vi "Read From String Format.vi"(8 "error in (no error)":errorcluster, 11 "Numeric in":refnum<class "Abs_Numeric_1D.lvclass">) -> (0 "error out":errorcluster, 2 "From String Format":string="%f", 3 "Numeric out":refnum<class "Abs_Numeric_1D.lvclass">)   [LabVIEW 2021, in "Abs_Numeric_1D.lvclass"]
uses:
  Abs_Numeric_1D.lvclass
  Abs_Numeric_1D.lvclass/Abs_Numeric_1D.ctl
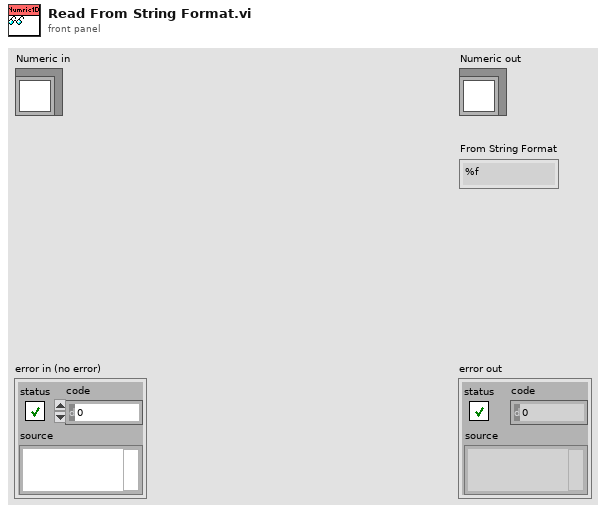
[diagram p1: front panel]
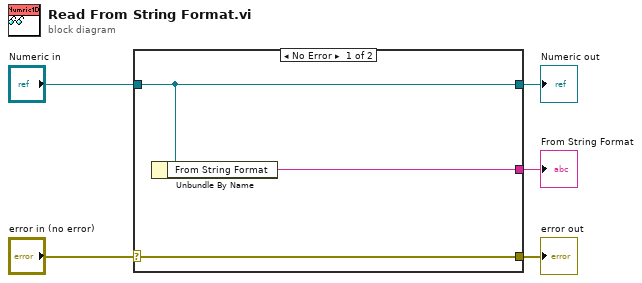
[diagram p0: block diagram]
diagram:
  n1 = case shown="No Error" "error in (no error)" {
    selector: "error in (no error)" -> [w8 w9]
    tunnel: [w8 w9] -> w4
    tunnel: [w7 w10] -> w2
    tunnel: "Numeric in" -> [w7 w10]
    tunnel: [w6 _] -> w1
    frame No Error {
      n2 = Unbundle By Name(w7) -> ("From String Format"=w6:string)
    }
    frame Error {
    }
  }
  "error out" <- w4
  "Numeric out" <- w2
  "From String Format" <- w1
